vi "DeQueue Trigger.vi"(0 "trigger queue in":refnum<queue>, 9 "timeout, ms (0)":i32, 11 "error in":errorcluster) -> (4 "trigger queue out":refnum<queue>, 6 "system trigger":T1, 10 "trigger data":variant, 15 "error out":errorcluster)   [LabVIEW 2015, in "TLB` Template.lvlib" / "{TMPL} Trigger API.lvlib"]
doc: "Removes an element from the front of a queue and returns the element.\n\n<B>Input Parameters</B>\n\n<B>trigger queue in</B> is a reference to a queue. Use the Create Trigger Queue function to obtain a queue reference. \n\n<B>timeout (ms)</B> trigger queue timeout.\n\n<B>error in</B> describes error conditions that occur before this node runs. This input provides standard error in functionality.\n\n<B>Output Parameters</B>\n\n<B>trigger queue</B> returns the reference to the queue unchanged. \n\n<B>system trigger</B> available system triggers.\n\n<B>trigger data</B> data message as part of the system trigger.\n\n<B>error out</B> contains error information. This output provides standard error out functionality."
uses:
  {TMPL} Trigger API.lvlib
  System Trigger.ctl
  System Trigger Element.ctl
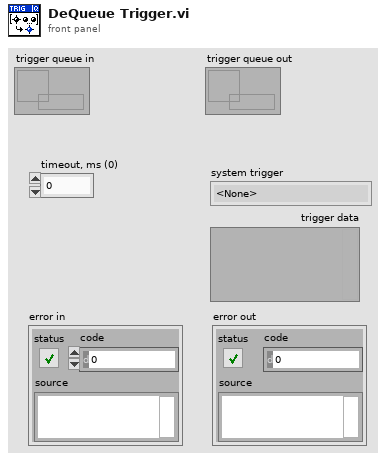
[diagram p1: front panel]
types:
  T1 = typedef "TLB` Template.lvlib/{TMPL} Trigger API.lvlib/System Trigger.ctl" = enum16{"<None>", "Connect", "Start Acquisition", "Stop Acquisition", "Disconnect", "<Return to Safe State Actions>", "<Cache User Parameters>", "<Close Application>", "<Error>"}
  T2 = typedef "TLB` Template.lvlib/{TMPL} Trigger API.lvlib/System Trigger Element.ctl" = cluster{"System Trigger":T1, "Trigger Data":variant}
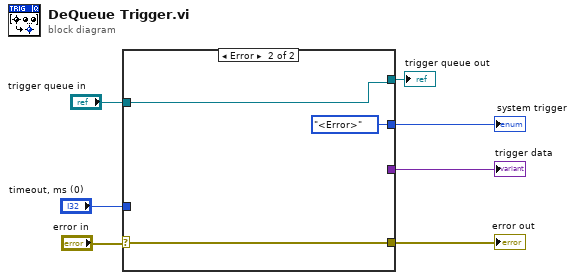
[diagram p0: block diagram]
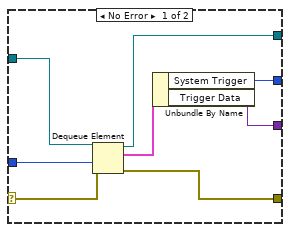
[diagram p2: hidden frame]
diagram:
  n1 = case shown="Error" "error in" {
    selector: "error in" -> [w10 w18]
    tunnel: [w15 w16] -> w1
    tunnel: [w14 w18] -> w7
    tunnel: "timeout, ms (0)" -> [w13 _]
    tunnel: [w8 System_Trigger."<Error>" ("System Triggers")] -> w2
    tunnel: [w11 _] -> w5
    tunnel: "trigger queue in" -> [w9 w16]
    frame No Error {
      n2 = Dequeue Element(queue=w9, timeout in ms (-1)=w13, error in (no error)=w10) -> (queue out=w15:refnum<queue>, element=w12:T2, error out=w14:errorcluster)  [unwired: 1 out]
      n3 = Unbundle By Name(w12) -> ("System Trigger"=w8:T1, "Trigger Data"=w11:variant)
    }
    frame Error {
    }
  }
  "system trigger" <- w2
  "error out" <- w7
  "trigger data" <- w5
  "trigger queue out" <- w1
